vi "SigArrayInit.vi"(0 "Signal Array":dbl[](array[numeric]), 1 "Pstat":refnum<k7>, 2 "Signal In":refnum<k7>, 5 "CtrlMode":u32, 7 "Cycles":i32, 9 "Sample Rate":dbl, 11 "error in (no error)":errorcluster) -> (4 "Pstat Out":refnum<k7>, 6 "Signal Out":refnum<k7>, 15 "error out":errorcluster)   [LabVIEW 2016]
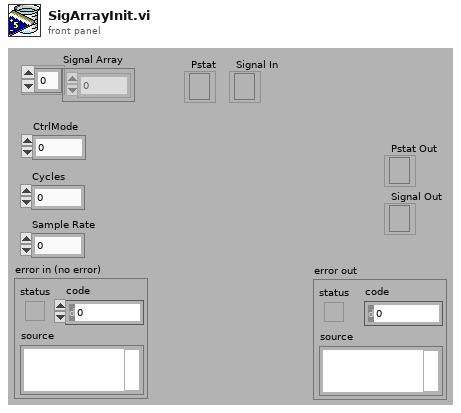
[diagram p1: front panel]
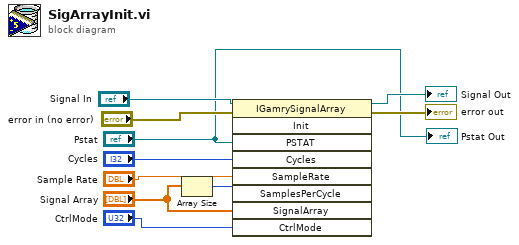
[diagram p0: block diagram]
diagram:
  n1 = Array Size(array="Signal Array") -> (size(s)=w4:i32)
  n2 = invoke class="IGamrySignalArray" method="Init"(reference="Signal In", error in="error in (no error)", "PSTAT"="Pstat", "Cycles"="Cycles", "SampleRate"="Sample Rate", "SamplesPerCycle"=w4, "SignalArray"="Signal Array", "CtrlMode"="CtrlMode") -> (reference out=→"Signal Out":refnum<k7>, error out=→"error out":errorcluster)  [unwired: 1 in, 7 out]
  "Pstat Out" <- "Pstat"
